vi "SensorDiagnosticsResult_SM.vi"(8 "error in (no error)":errorcluster, 10 "ImagesAndCount":cluster{"Image Array":T1[], "ImageCount":u64}, 11 "Inspection Statemachine in":refnum<class "Inspection Statemachine.lvclass">) -> (0 "error out":errorcluster, 3 "Inspection Statemachine out":refnum<class "Inspection Statemachine.lvclass">)   [LabVIEW 2019, in "Inspection Statemachine.lvclass"]
uses:
  Inspection Statemachine.lvclass
  <vilib>/vision/Image Controls.llb/IMAQ Image.ctl
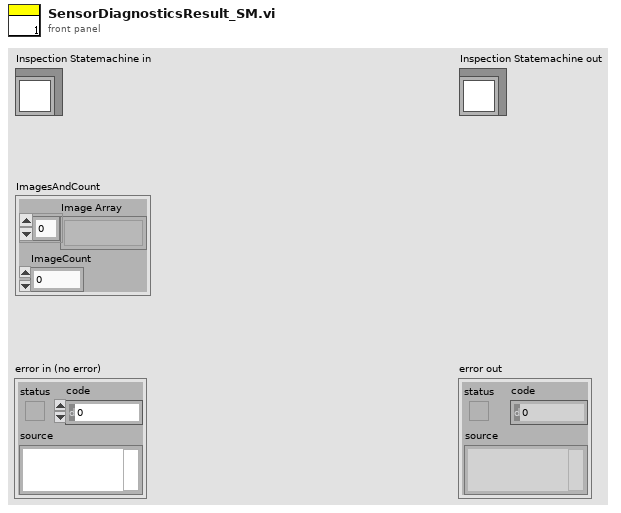
[diagram p1: front panel]
types:
  T1 = typedef "IMAQ Image.ctl" = refnum<image>
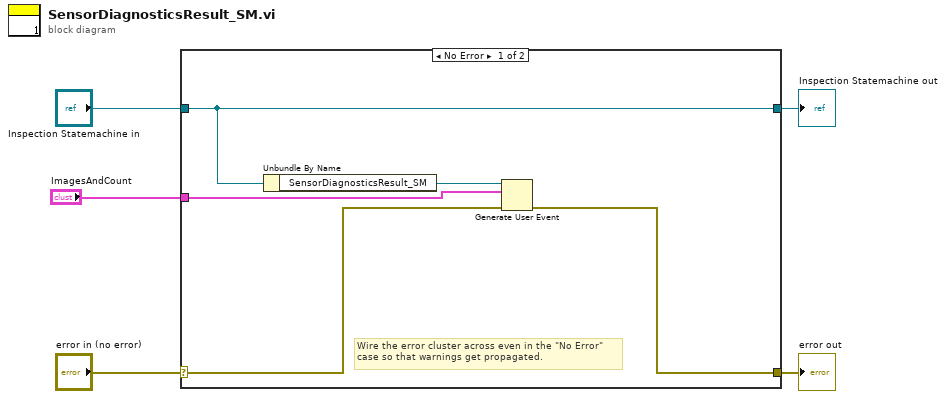
[diagram p0: block diagram]
diagram:
  n1 = case shown="No Error" "error in (no error)" {
    selector: "error in (no error)" -> [w8 w12]
    tunnel: [w7 w12] -> w4
    tunnel: [w10 w11] -> w2
    tunnel: "Inspection Statemachine in" -> [w10 w11]
    tunnel: "ImagesAndCount" -> [w6 _]
    frame No Error {
      # "Wire the error cluster across even in the \"No Error\"\ncase so that warnings get propagated."
      n2 = Unbundle By Name(w10) -> ("SensorDiagnosticsResult_SM"=w9:refnum<user-event>)
      n3 = Generate User Event(user event=w9, event data cluster=w6, error in=w8) -> (error out=w7:errorcluster)  [unwired: 1 in, 1 out]
    }
    frame Error {
    }
  }
  "error out" <- w4
  "Inspection Statemachine out" <- w2
